vi "CastlingUpdate.vi"(1 "L/R (T/F)":bool, 2 "Black/White Turn (T/F)":bool, 3 "Castling State":bool[][](array[boolean])=[[TRUE, TRUE, TRUE], [TRUE, TRUE, TRUE]]) -> (0 "Update Castling State":bool[][](array[boolean]))   [LabVIEW 2014]
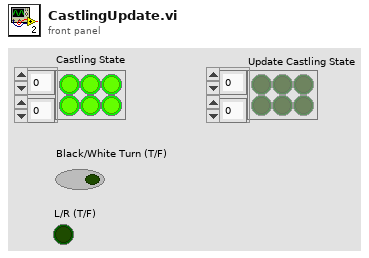
[diagram p1: front panel]
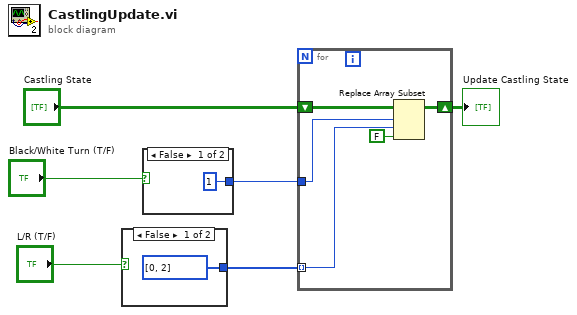
[diagram p0: block diagram]
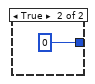
[diagram p2: hidden frame]
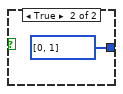
[diagram p3: hidden frame]
diagram:
  n1 = case shown="False" "L/R (T/F)" {
    tunnel: [i32[] [0, 2] i32[] [0, 1]] -> w3
    frame False {
    }
    frame True {
    }
  }
  n2 = case shown="False" "Black/White Turn (T/F)" {
    tunnel: [1 0] -> w2
    frame False {
    }
    frame True {
    }
  }
  n3 = for {
    tunnel: w3 -> [w13] mode=indexing
    tunnel: w2 -> [w14]
    shift-right: [w11] -> w1
    shift-left: "Castling State" -> [w15]
    n4 = Replace Array Subset(array=w15, new element=FALSE ("new element/subarray"), index (row)=w14, index (col)=w13) -> (w11:bool[][])
  }
  "Update Castling State" <- w1
